vi "Display logs.vi"(8 "error in (no error)":errorcluster, 11 "Logger in":refnum<class "Logger.lvclass">) -> (0 "error out":errorcluster, 2 "Display":string, 3 "Logger out":refnum<class "Logger.lvclass">)   [LabVIEW 2017, in "Logger.lvclass"]
uses:
  Logger.lvclass
  Logger.lvclass/Logger.ctl
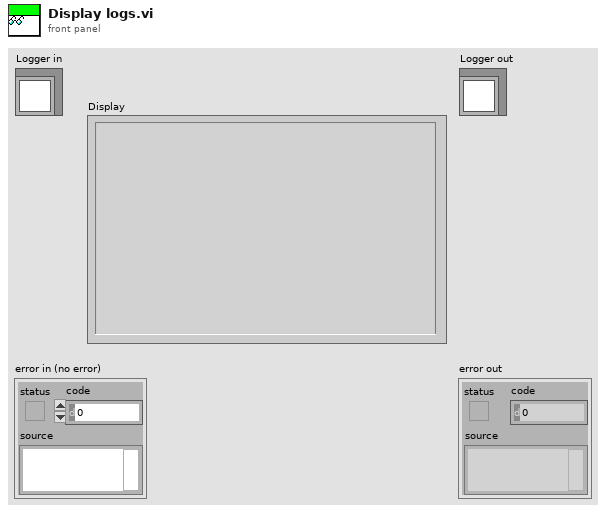
[diagram p1: front panel]
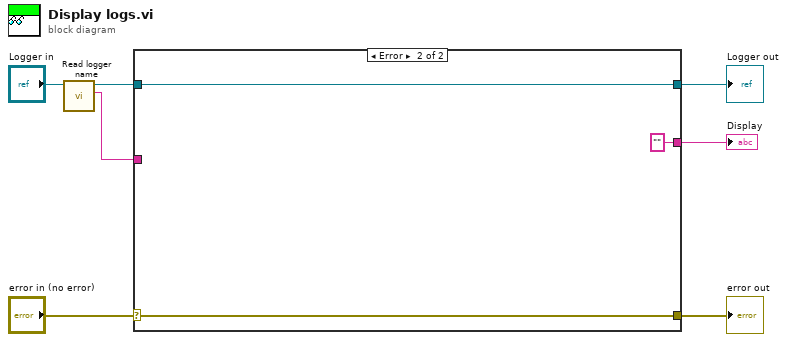
[diagram p0: block diagram]
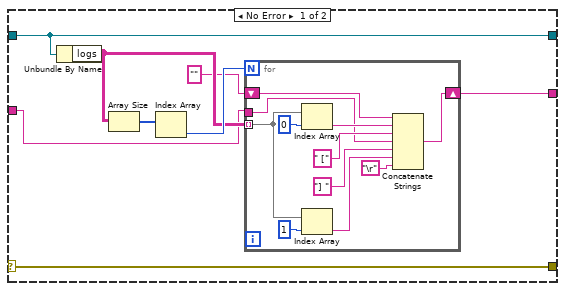
[diagram p2: hidden frame]
diagram:
  n1 = call-dynamic "Read logger name.vi"("Logger in"="Logger in") -> ("logger name"=w2:string, "Logger out"=w4:refnum<class "Logger.lvclass">)  [unwired: 9 in]
  n2 = case shown="Error" "error in (no error)" {
    selector: "error in (no error)" -> [w15 w28]
    tunnel: [w15 w28] -> w6
    tunnel: [w14 w29] -> w5
    tunnel: w4 -> [w14 w29]
    tunnel: w2 -> [w10 _]
    tunnel: [w8 ""] -> w1
    frame No Error {
      n3 = Unbundle By Name(w14) -> ("logs"=w11:string[][])
      n4 = Array Size(array=w11) -> (size(s)=w13:i32[])
      n5 = Index Array(array=w13) -> (element=w12:i32)  [unwired: 1 in]
      n6 = for {
        N: w12 -> [_]
        tunnel: w11 -> [w26] mode=indexing
        tunnel: w10 -> [w22]
        shift-right: [w16] -> w8
        shift-left: "" -> [w24]
        n7 = Index Array(array=w26, index=0) -> (element=w25:string)
        n8 = Index Array(array=w26, index=1) -> (element=w20:string)
        n9 = Concatenate Strings(w24, w25, " [" ("string"), w22, "] " ("string"), w20, "\r") -> (w16:string)
      }
    }
    frame Error {
    }
  }
  "error out" <- w6
  "Logger out" <- w5
  "Display" <- w1
